vi "Close.vi"(8 "error in (no error)":errorcluster, 11 "NhRegenGridSim in":refnum<class "NHRGridSim.lvclass">) -> (0 "error out":errorcluster, 3 "NhRegenGridSim out":refnum<class "NHRGridSim.lvclass">)   [LabVIEW 2018, in "AcPwrPlugins.lvlib" / "NHRGridSim.lvclass"]
doc: "This VI closes the connection to the instrument(s)."
uses:
  NHRGridSim.lvclass
  <instrlib>/NH Research 9400 Series/NH Research 9400 Series.lvlib
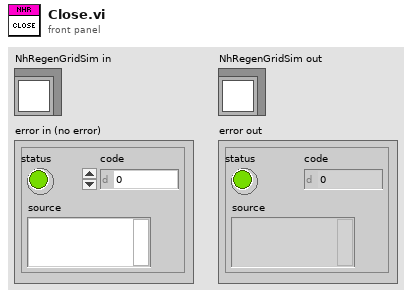
[diagram p1: front panel]
types:
  T1 = typedef "AcPwrPlugins.lvlib/NHRGridSim.lvclass/NHRGrid_Device(s)Settings.ctl" = cluster{"MeasName":string, "Hardware":T2}
  T2 = typedef "AcPwrPlugins.lvlib/NHRGridSim.lvclass/NHRGrid_Hardware.ctl" = cluster{"Handle":string, "Reset":bool, "Mode":T3, "ID Query":bool, "Logical Instrument":T4, "Connected":bool}
  T3 = typedef "AcPwrPlugins.lvlib/NHRGridSim.lvclass/NHRGrid_Modes.ctl" = u8
  T4 = typedef "AcPwrPlugins.lvlib/NHRGridSim.lvclass/NHRGrid_Logical_Instrument.ctl" = cluster{"Name":string, "Vout (V)":dbl, "I limit (A)":dbl, "P limit (W)":dbl, "FreqOut (Hz)":dbl, "Ranges":cluster{"Voltage (V)":u16, "Current (A)":u16}, "Configure Instrument":u16, "Aperture (cycles)":i32, "AC Wave Shape":u16, "VType":string, "IType":string, "Phases":T5, "Slew Rates":T6, "Safety Trips":T7}[]
  T5 = typedef "AcPwrPlugins.lvlib/NHRGridSim.lvclass/NHRGrid_Phases.ctl" = cluster{"A-Volts (V)":dbl, "B-Volts (V)":dbl, "C-Volts (V)":dbl, "A-Curr (A)":dbl, "B-Curr (A)":dbl, "C-Curr (A)":dbl, "A-Power (W)":dbl, "B-Power (W)":dbl, "C-Power (W)":dbl, "Change at (Deg)":dbl, "B-Angle (Deg)":dbl, "C-Angle (Deg)":dbl}
  T6 = typedef "AcPwrPlugins.lvlib/NHRGridSim.lvclass/NHRGrid_SlewRates.ctl" = cluster{"Vmax (V/s)":dbl, "Vmin (V/s)":dbl, "Imax (A/s)":dbl, "Imin (A/s)":dbl, "Pmax (W/s)":dbl, "Pmin (W/s)":dbl, "Freq Max (Hz/s)":dbl, "Freq Min (Hz/s)":dbl, "Phase Angle Max (Deg/s)":dbl, "Phase Angle Min (Deg/s)":dbl}
  T7 = typedef "AcPwrPlugins.lvlib/NHRGridSim.lvclass/NHRGrid_SafetyTrips.ctl" = cluster{"Vmax (V)":dbl, "Vmin (V)":dbl, "Vmax Time (s)":dbl, "Vmin Time (s)":dbl, "Imax Source (A)":dbl, "Imax Sink (A)":dbl, "Imax Source Time (s)":dbl, "Imax Sink Time (s)":dbl, "Pmax Source (W)":dbl, "Pmax Sink (W)":dbl, "Pmax Source Time (s)":dbl, "Pmax Sink Time (s)":dbl, "Absolute Volt Peak":dbl, "Enable Volt Peak":bool, "Absolute Curr Peak":dbl, "Enable Curr Peak":bool}
  T8 = typedef "AcPwrPlugins.lvlib/NHRGridSim.lvclass/Measurements.ctl" = cluster{"Handle":string, "Name":string, "Enabled ":bool, "Measurement Value":dbl, "Instrument Number ":i32, "Measurement Type ":T9}[]
  T9 = typedef "AcPwrPlugins.lvlib/NHRGridSim.lvclass/MeasurementType.ctl" = enum16{"Average Current", "Average Voltage"}
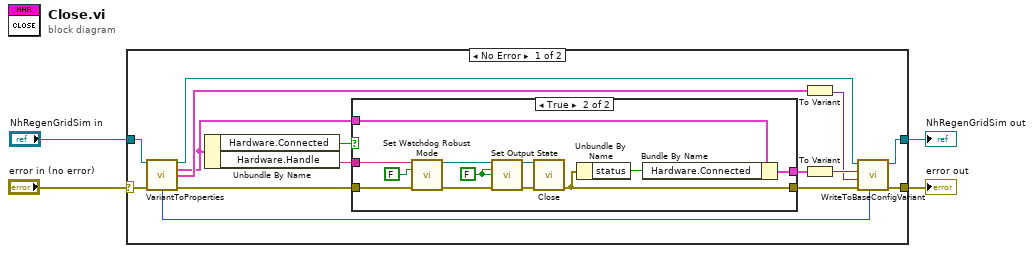
[diagram p0: block diagram]
diagram:
  n1 = case shown="No Error" "error in (no error)" {
    selector: "error in (no error)" -> [w18 w34]
    tunnel: "NhRegenGridSim in" -> [w17 w35]
    tunnel: [w15 w35] -> w3
    tunnel: [w14 w34] -> w2
    frame No Error {
      n2 = call "VariantToProperties.vi"("NHRGridSim in"=w17, "error in (no error)"=w18) -> ("NHRGridSim out"=w16:refnum<class "NHRGridSim.lvclass">, "Device(s)Settings"=w11:T1, "Measurements"=w13:T8, "Measurement Refresh Time (ms)"=w12:u32, "error out"=w19:errorcluster)  [unwired: 8 in, 1 out]
      n3 = Unbundle By Name(w11) -> ("Hardware.Connected"=w6:bool, "Hardware.Handle"=w7:string)
      n4 = case shown="True" w6 {
        tunnel: [w21 w31] -> w9
        tunnel: w19 -> [w21 w29]
        tunnel: w7 -> [_ w28]
        tunnel: w11 -> [w20 w33]
        tunnel: [w20 w32] -> w5
        frame False {
        }
        frame True {
          w22 = FALSE ("Robust Mode (F: Disable)")
          n5 = call <instrlib>:"Set Watchdog Robust Mode.vi"("VISA resource name"=w28, "Robust Mode (F: Disable)"=FALSE, "error in (no error)"=w29) -> ("VISA resource name out"=w26:refnum<visa-resource-name>, "error out"=w27:errorcluster)  [unwired: 11 in]
          n6 = call <instrlib>:"Set Output State.vi"("VISA resource name"=w26, "Output State (F: Disable)"=w22, "All (F: Disable)"=w22, "error in (no error)"=w27) -> ("VISA resource name out"=w24:refnum<visa-resource-name>, "error out"=w25:errorcluster)  [unwired: 10 in]
          n7 = call <instrlib>:"Close.vi"("VISA resource name"=w24, "error in (no error)"=w25) -> ("error out"=w31:errorcluster)  [unwired: 13 in]
          n8 = Unbundle By Name(w31) -> ("status"=w30:bool)
          n9 = Bundle By Name(cluster=w33, "Hardware.Connected"=w30) -> (w32:T1)
        }
      }
      n10 = To Variant(anything=w13) -> (Variant=w8:variant)
      n11 = To Variant(anything=w5) -> (Variant=w10:variant)
      n12 = call "WriteToBaseConfigVariant.vi"("Measurement RefreshTime (ms)"=w12, "error in (no error)"=w9, "Meas"=w8, "Config"=w10, "NHRGridSim in"=w16) -> ("error out"=w14:errorcluster, "NHRGridSim out"=w15:refnum<class "NHRGridSim.lvclass">)  [unwired: 5 in]
    }
    frame Error {
    }
  }
  "error out" <- w2
  "NhRegenGridSim out" <- w3
